vi "RotateAll.vi"() -> ()   [LabVIEW 2017]
panel:
  in  "Reference Frame":i32=5000
  out "Horizontal Progress Bar":u8(slide) scale=0.0..2.0
  out "Rotating":dbl
  out "Total Video Segments to Rotate":dbl
  # "This VI rotates all AVI videos in the selected folder. The user is prompted to select the folder after which they are asked to draw a line in the middle of the vessel (bottom to top). The program will then run autonomously to rotate all the videos such as the vessel is horizontal."
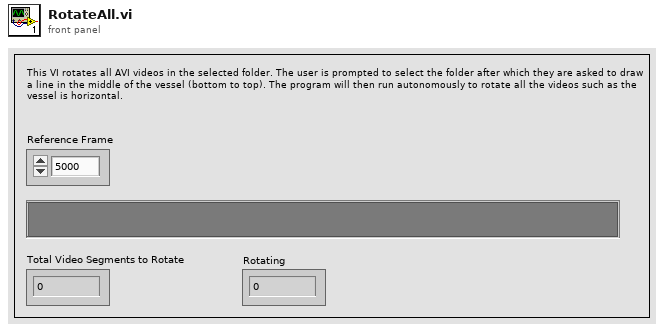
[diagram p1: front panel]
types:
  T1 = typedef "IMAQ AVI2 Refnum.ctl" = refnum<k20>
  T2 = typedef "IMAQ Image.ctl" = refnum<image>
  T3 = typedef "IMAQ Line" = cluster{"Start X":i32, "Start Y":i32, "End X":i32, "End Y":i32}
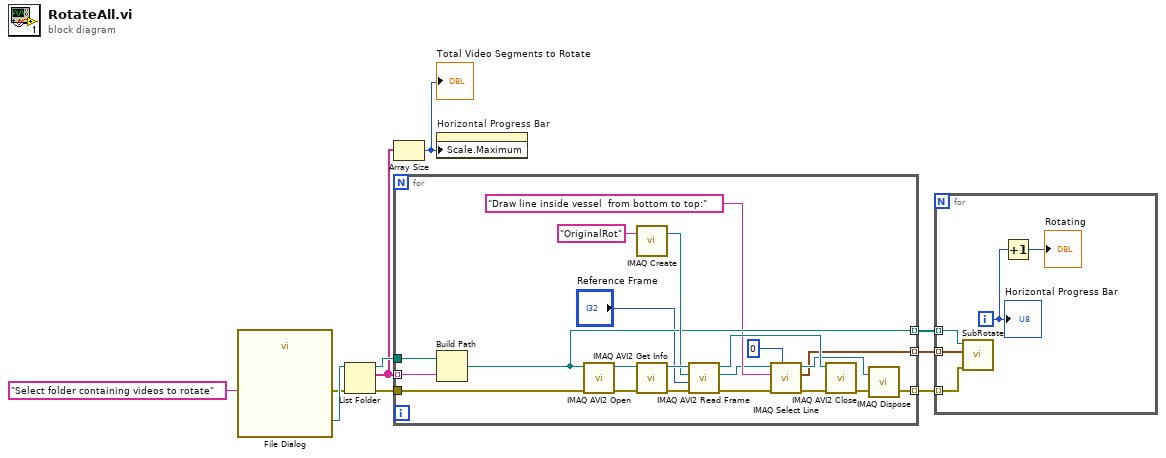
[diagram p0: block diagram]
diagram:
  n1 = call "File Dialog"("prompt"="Select folder containing videos to rotate") -> ("selected path"=w9:path, "error out"=w8:errorcluster)  [unwired: 11 in, 2 out]
  n2 = List Folder(path=w9, error in=w8) -> (path out=w7:path, filenames=w3:string[], error out=w6:errorcluster)  [unwired: 2 in, 1 out]
  n3 = Array Size(array=w3) -> (size(s)=w2:i32)
  "Total Video Segments to Rotate" <- w2
  n4 = for {
    tunnel: w7 -> [w31]
    tunnel: w3 -> [w30] mode=indexing
    tunnel: w6 -> [w23]
    tunnel: [w19] -> w5 mode=indexing
    tunnel: [w21] -> w4 mode=indexing
    tunnel: [w12] -> w1 mode=indexing
    n5 = Build Path(base path=w31, name or relative path=w30) -> (appended path=w21:path)
    n6 = call "IMAQ AVI2 Open"("error in (no error)"=w23, "AVI File Path"=w21) -> ("error out"=w28:errorcluster, "AVI Refnum"=w29:T1)  [unwired: 8 in]
    n7 = call "IMAQ Create"("Image Name"="OriginalRot") -> ("New Image"=w25:T2)  [unwired: 4 in, 1 out]
    n8 = call "IMAQ AVI2 Get Info"("error in (no error)"=w28, "AVI Refnum"=w29) -> ("error out"=w24:errorcluster, "AVI Refnum (duplicate)"=w27:T1)  [unwired: 5 in, 3 out]
    n9 = call "IMAQ AVI2 Read Frame"("error in (no error)"=w24, "Frame Number"="Reference Frame", "Image"=w25, "AVI Refnum"=w27) -> ("error out"=w15:errorcluster, "Image Out"=w17:T2, "AVI Refnum (duplicate)"=w22:T1)  [unwired: 5 in]
    n10 = call "IMAQ Select Line"("Window Number (0...15)"=0, "error in (no error)"=w15, "Prompt"="Draw line inside vessel  from bottom to top:", "Image In"=w17) -> ("error out"=w14:errorcluster, "Line"=w12:T3, "Image Out (duplicate)"=w13:T2)  [unwired: 4 in, 1 out]
    n11 = call "IMAQ AVI2 Close"("error in (no error)"=w14, "AVI Refnum"=w22) -> ("error out"=w20:errorcluster)  [unwired: 9 in]
    n12 = call "IMAQ Dispose"("Image"=w13, "error in (no error)"=w20) -> ("error out"=w19:errorcluster)  [unwired: 4 in]
  }
  n13 = property on="Horizontal Progress Bar" class="Slide (strict)"("Scale.Maximum"=w2) -> ()  [unwired: 2 in, 2 out]
  n14 = for {
    tunnel: w5 -> [w34] mode=indexing
    tunnel: w4 -> [w36] mode=indexing
    tunnel: w1 -> [w35] mode=indexing
    i -> [w32]
    n15 = call "SubRotate.vi"("error in (no error)"=w34, "input cluster"=w35, "AVI Path"=w36) -> ()  [unwired: 8 in, 1 out]
    n16 = Increment(x=w32) -> (x+1=→"Rotating":i32)
    "Horizontal Progress Bar" <- w32
  }
